vi "Read Ref Value.vi"(8 "error in (no error)":errorcluster, 11 "BetterBoxHandle in":refnum<class "BetterBoxHandle.lvclass">) -> (0 "error out":errorcluster, 2 "Value":i32[](array[numeric]), 3 "BetterBoxHandle out":refnum<class "BetterBoxHandle.lvclass">)   [LabVIEW 2020, in "BetterDragAndDrop.lvlib" / "BetterBoxHandle.lvclass"]
uses:
  BetterBoxHandle.lvclass
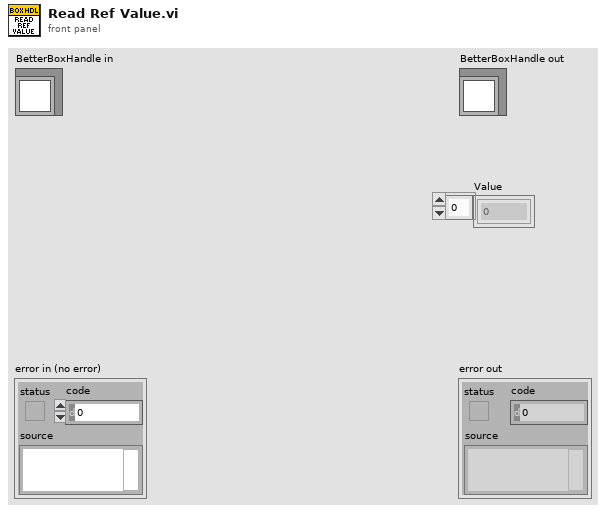
[diagram p1: front panel]
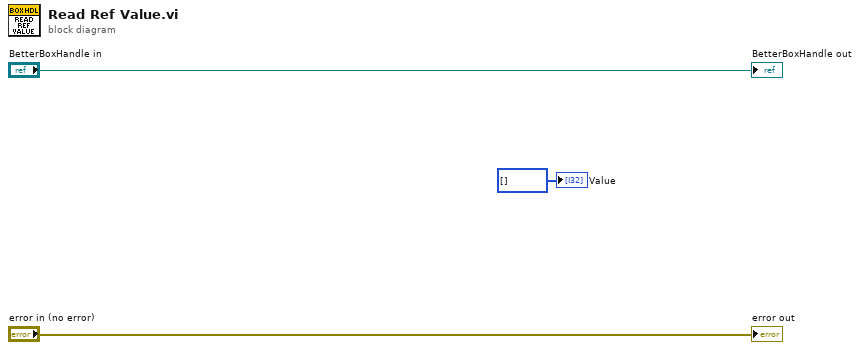
[diagram p0: block diagram]
diagram:
  "error out" <- "error in (no error)"
  "BetterBoxHandle out" <- "BetterBoxHandle in"
  "Value" <- i32[] [] ("Value")
